vi "create_DSCEvent.vi"(0 "Host_Reference":refnum<class "HGF_Reference.lvclass">, 2 "timeout in ms (-1)":i32=-1, 5 "error in (no error)":errorcluster) -> (14 "dup Host_Reference":refnum<class "HGF_Reference.lvclass">, 19 "error out":errorcluster)   [LabVIEW 2009, in "MoAgSy.lvlib" / "MoAgSy_Host.lvclass"]
doc: "<B>public</B> VI reads DSC settings and creates a new DSC Event that waits for an incoming string at Host Variable. The Event is part of the hosts communication interface.\n\nF.Berck@gsi.de\nGSI Darmstadt 2009"
uses:
  MoAgSy_Host.lvclass
  HGF_BaseClasses/HGF_Reference/HGF_Reference.lvclass
  HGF_BaseClasses/HGF_Event/HGF_Event.lvclass
  HGF_DSC/HGF_DSCEvent/HGF_DSCEvent.lvclass
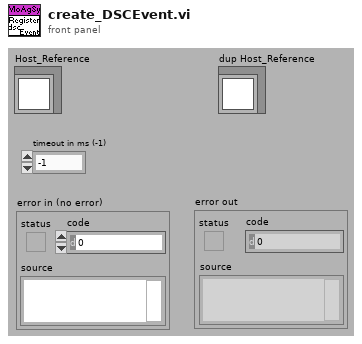
[diagram p1: front panel]
types:
  T1 = cluster{"Host Variable":refnum<k21>, "Agent_Event (Monitor Event)":refnum<class "HGF_Event.lvclass">, "Host_Event (Monitor Event)":refnum<class "HGF_Event.lvclass">, "DSCException":refnum<class "HGF_TriggeredEvent.lvclass">, "MoAgSy_DSCThreadPool":refnum<class "HGF_Reference.lvclass">, "ManagerEvent":refnum<class "HGF_Event.lvclass">, "DSCDestination":refnum<class "HGF_TriggeredEvent.lvclass">}
  T2 = cluster{"DSC Event":refnum<class "HGF_Event.lvclass">}
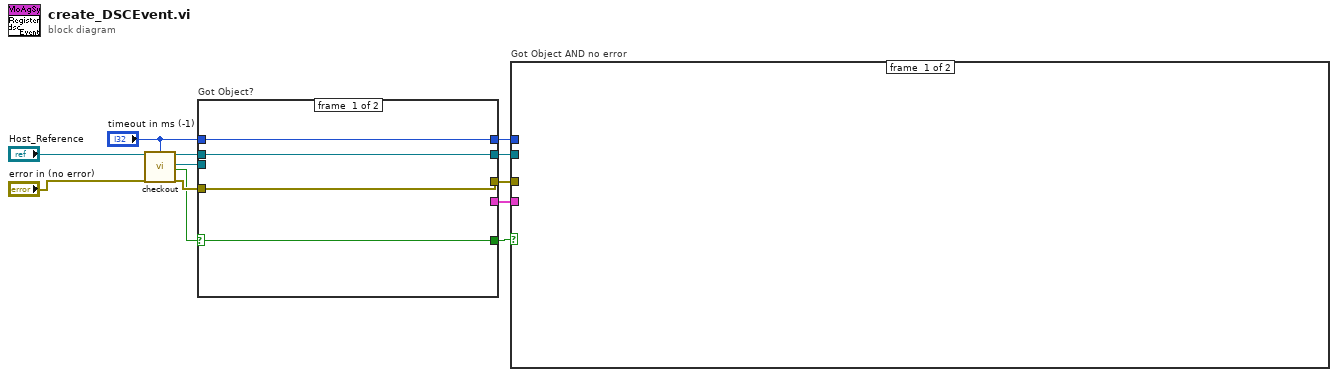
[diagram p0: block diagram]
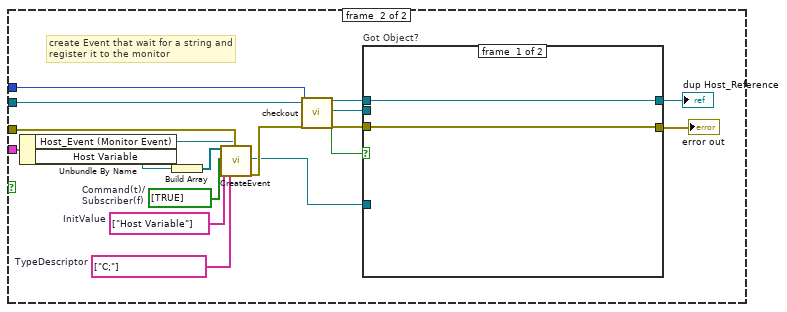
[diagram p2: hidden frame]
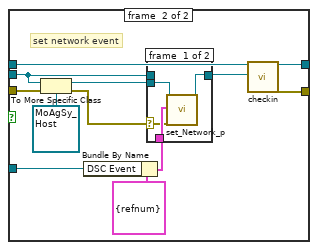
[diagram p3: hidden frame]
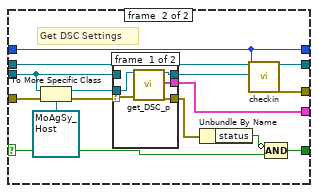
[diagram p5: hidden frame]
diagram:
  n1 = call "checkout.vi"("HGF_Reference"="Host_Reference", "timeout in ms (-1)"="timeout in ms (-1)", "error in (no error)"="error in (no error)") -> ("dup HGF_Reference"=w7:refnum<class "HGF_Reference.lvclass">, "Object"=w8:refnum<class>, "got object?"=w9:bool, "error out"=w10:errorcluster)  [unwired: 13 out]
  n2 = case "Got Object?" shown="True" w9 {
    selector: w9 -> [w13 w18]
    tunnel: w8 -> [_ w21]
    tunnel: w7 -> [w16 w31]
    tunnel: [w16 w30] -> w3
    tunnel: "timeout in ms (-1)" -> [w14 w24]
    tunnel: [w15 w29] -> w4
    tunnel: w10 -> [w15 w28]
    tunnel: [_ w26] -> w5
    tunnel: [w14 w24] -> w2
    tunnel: [w13 w19] -> w1
    frame #0 {
    }
    frame #1 {
      # "Get DSC Settings"
      n3 = To More Specific Class(target class=refnum<class "MoAgSy_Host.lvclass"> refnum ("MoAgSy.lvlib:MoAgSy_Host.lvclass"), reference=w21, error in=w28) -> (specific class reference=w25:refnum<class "MoAgSy_Host.lvclass">, error out=w22:errorcluster)
      n4 = case shown="No Error" w22 {
        selector: w22 -> [w32 _]
        tunnel: [w36 w37] -> w27
        tunnel: [w35 _] -> w20
        tunnel: [w34 _] -> w26
        tunnel: w25 -> [w33 _]
        tunnel: w21 -> [_ w37]
        frame #0 {
          n5 = call "get_DSC_p.vi"("MoAgSy_Host"=w33, "error in (no error)"=w32) -> ("dup MoAgSy_Host"=w36:refnum<class "MoAgSy_Host.lvclass">, "DSC"=w34:T1, "error out"=w35:errorcluster)  [unwired: 15 out]
        }
        frame #1 {
        }
      }
      n6 = Unbundle By Name(w20) -> ("status"=w17:bool)
      n7 = call "checkin.vi"("HGF_Reference"=w31, "Object"=w27, "timeout /ms (-1)"=w24) -> ("dup HGF_Reference"=w30:refnum<class "HGF_Reference.lvclass">, "error out"=w29:errorcluster)  [unwired: 1 in, 14 out]
      n8 = Compound Arithmetic op=AND(invert w17, w18) -> (w19:bool)
    }
  }
  n9 = case "Got Object AND no error" shown="True" w1 {
    tunnel: w5 -> [_ w55]
    tunnel: w4 -> [_ w51]
    tunnel: w3 -> [_ w50]
    tunnel: w2 -> [_ w48]
    frame #0 {
    }
    frame #1 {
      w39 = string[] ["Host Variable"]  # InitValue
      w40 = string[] ["C;"]  # TypeDescriptor
      w52 = bool[] [TRUE]  # Command(t)/ Subscriber(f)
      # "create Event that wait for a string and\nregister it to the monitor"
      n10 = Unbundle By Name(w55) -> ("Host_Event (Monitor Event)"=w38:refnum<class "HGF_Event.lvclass">, "Host Variable"=w54:refnum<k21>)
      n11 = Build Array(w54) -> (w53:refnum<k21>[])
      n12 = call "CreateEvent.vi"("Shared Variable"=w53, "TypeDescriptor"=w40, "Command(t)/\nSubscriber(f)"=w52, "InitValue"=w39, "error in (no error)"=w51, "HGF_Event (Monitor Event)"=w38) -> ("HGF Event"=w41:refnum<class "HGF_Event.lvclass">, "error out"=w49:errorcluster)  [unwired: 12 in]
      n13 = call "checkout.vi"("HGF_Reference"=w50, "timeout in ms (-1)"=w48, "error in (no error)"=w49) -> ("dup HGF_Reference"=w45:refnum<class "HGF_Reference.lvclass">, "Object"=w46:refnum<class>, "got object?"=w47:bool, "error out"=w44:errorcluster)  [unwired: 13 out]
      n14 = case "Got Object?" shown="True" w47 {
        tunnel: [w57 w68] -> w42
        tunnel: [w56 w67] -> w43
        tunnel: w46 -> [_ w58]
        tunnel: w45 -> [w57 w66]
        tunnel: w44 -> [w56 w65]
        tunnel: w41 -> [_ w60]
        frame #0 {
        }
        frame #1 {
          # "set network event"
          n15 = To More Specific Class(target class=refnum<class "MoAgSy_Host.lvclass"> refnum ("MoAgSy.lvlib:MoAgSy_Host.lvclass"), reference=w58, error in=w65) -> (specific class reference=w64:refnum<class "MoAgSy_Host.lvclass">, error out=w59:errorcluster)
          n16 = Bundle By Name(cluster=T2 {"DSC Event"=refnum} ("Network"), "DSC Event"=w60) -> (w61:T2)
          n17 = case shown="No Error" w59 {
            selector: w59 -> [w70 _]
            tunnel: w64 -> [w73 _]
            tunnel: [w72 w74] -> w63
            tunnel: w61 -> [w71 _]
            tunnel: w58 -> [_ w74]
            frame #0 {
              n18 = call "set_Network_p.vi"("MoAgSy_Host"=w73, "Network"=w71, "error in (no error)"=w70) -> ("dup MoAgSy_Host"=w72:refnum<class "MoAgSy_Host.lvclass">)  [unwired: 16 out]
            }
            frame #1 {
            }
          }
          n19 = call "checkin.vi"("HGF_Reference"=w66, "Object"=w63) -> ("dup HGF_Reference"=w68:refnum<class "HGF_Reference.lvclass">, "error out"=w67:errorcluster)  [unwired: 2 in, 14 out]
        }
      }
      "dup Host_Reference" <- w42
      "error out" <- w43
    }
  }
